vi "Handle Error.vi"(8 "error in (no error)":errorcluster, 11 "LoggedActor in":refnum<class "LoggedActor.lvclass">) -> (0 "error out":errorcluster, 2 "stop actor?":bool=TRUE, 3 "LoggedActor out":refnum<class "LoggedActor.lvclass">)   [LabVIEW 2019, in "LoggedActor.lvclass"]
doc: "(<B>Filename</B>: Actor Framework.lvlib:Actor.lvclass:Handle Error.vi)\n\nDefines how the actor handles an error that occurred while processing a message. By default, this method does nothing except stop the actor."
uses:
  <vilib>/gpm_packages/@cs/Network-interface/Source/Logged Actor/LoggedActor.lvclass
  <vilib>/gpm_packages/@cs/event-logger/Source/Composed Log/Types/Log Level.ctl
  <vilib>/gpm_packages/@cs/Network-interface/Source/Logged Actor/LoggedActor.lvclass/LoggedActor.ctl
  <vilib>/gpm_packages/@cs/event-logger/Source/Composed Log/LoggerReference/LoggerReference.lvclass/LoggerReference.ctl
  <vilib>/gpm_packages/@cs/event-logger/Source/Composed Log/LoggerReference/Log Event.vi
  <vilib>/gpm_packages/@cs/event-logger/Source/Composed Log/LoggerReference/Log.vi
  <vilib>/gpm_packages/@cs/event-logger/Source/Composed Log/LoggerReference/Get Valid Event Time.vi
  <vilib>/gpm_packages/@cs/event-logger/Source/Composed Log/LoggerReference/Remove Stale Logs.vi
  <vilib>/ActorFramework/Actor/Actor.lvclass
  <vilib>/gpm_packages/@cs/event-logger/Source/Composed Log/Composed Log.lvlib
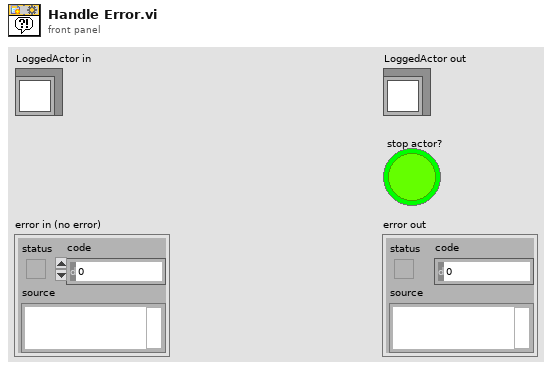
[diagram p1: front panel]
types:
  T1 = typedef "Composed Log.lvlib/Log Level.ctl" = enum16{"Debug", "Info", "Warning", "Error", "Critical"}
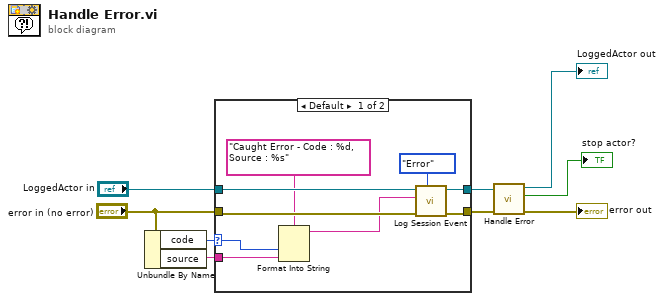
[diagram p0: block diagram]
diagram:
  n1 = Unbundle By Name("error in (no error)") -> ("code"=w5:i32, "source"=w1:string)
  n2 = case shown="Default" w5 {
    selector: w5 -> [w13 _]
    tunnel: "LoggedActor in" -> [w18 w20]
    tunnel: [w17 w20] -> w4
    tunnel: "error in (no error)" -> [w16 w19]
    tunnel: [w15 w19] -> w2
    tunnel: w1 -> [w12 _]
    frame Default {
      n3 = Format Into String(format string="Caught Error - Code : %d, Source : %s", w13, w12) -> (resulting string=w10:string)  [unwired: 2 in, 1 out]
      n4 = call <vilib>:"Log Session Event.vi"("Event Level"=Log_Level."Error", "error in (no error)"=w16, "Event Data"=w10, "SessionActor in"=w18) -> ("error out"=w15:errorcluster, "SessionActor out"=w17:refnum<class "LoggedActor.lvclass">)  [unwired: 6 in]
    }
    frame 0, 43, 1608 {
    }
  }
  n5 = call-parent "Handle Error.vi"("error in (no error)"=w2, "Actor in"=w4) -> ("error out"=→"error out":errorcluster, "stop actor?"=→"stop actor?":bool, "Actor out"=→"LoggedActor out":refnum<class "LoggedActor.lvclass">)  [unwired: 7 in]
